vi "PMBus Get Alert.vi"(7 "pAlertFlag":string, 8 "error in (no error)":errorcluster, 9 "PMBusIndex":i32, 10 "DevIndex":i32, 11 "DevType":i32) -> (0 "error out":errorcluster, 3 "function return":i32, 5 "pAlertFlag out":string)   [LabVIEW 2012, in "ControlPMBus.lvlib"]
doc: "int WINAPI PMBus_GetAlert(int DevType,int DevIndex,int PMBusIndex,unsigned char *pAlertFlag);"
uses:
  ControlPMBus.lvlib
  Ginkgo_Driver.dll
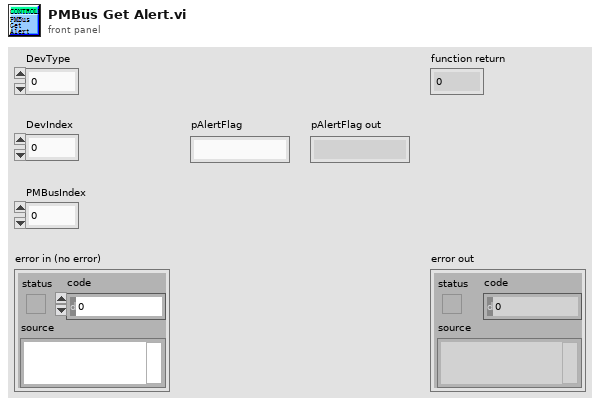
[diagram p1: front panel]
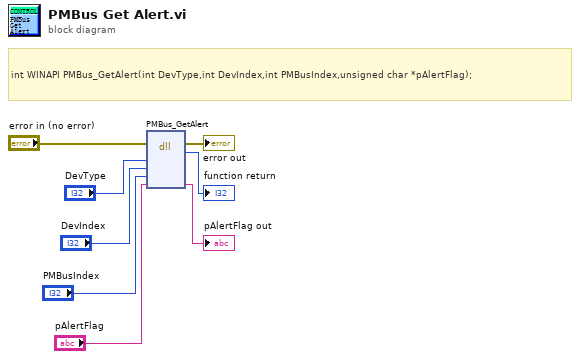
[diagram p0: block diagram]
diagram:
  # "int WINAPI PMBus_GetAlert(int DevType,int DevIndex,int PMBusIndex,unsigned char *pAlertFlag);"
  n1 = dll-call lib="E:/Project/vt_ginkgo/truck/Ginkgo Driver/vs2010/Ginkgo_USB-I2C_API_v2.0.3.0/lib/labview_64bit/ControlPMBus/Ginkgo_Driver.*" fn="PMBus_GetAlert"(error in="error in (no error)", "DevType"="DevType", "DevIndex"="DevIndex", "PMBusIndex"="PMBusIndex", "pAlertFlag"="pAlertFlag") -> (error out=→"error out":errorcluster, →"function return":i32, "pAlertFlag"=→"pAlertFlag out":string)  [unwired: 5 in, 1 out]
